vi "write_attributes.vi"(8 "error in (no error)":errorcluster, 10 "attributes":T1, 11 "GaussianNB in":refnum<class "GaussianNB.lvclass">) -> (0 "error out":errorcluster, 3 "GaussianNB out":refnum<class "GaussianNB.lvclass">)   [LabVIEW 2020, in "GaussianNB.lvclass"]
uses:
  GaussianNB.lvclass
  Controls/gaussian_nb_attributes.ctl
  GaussianNB.lvclass/GaussianNB.ctl
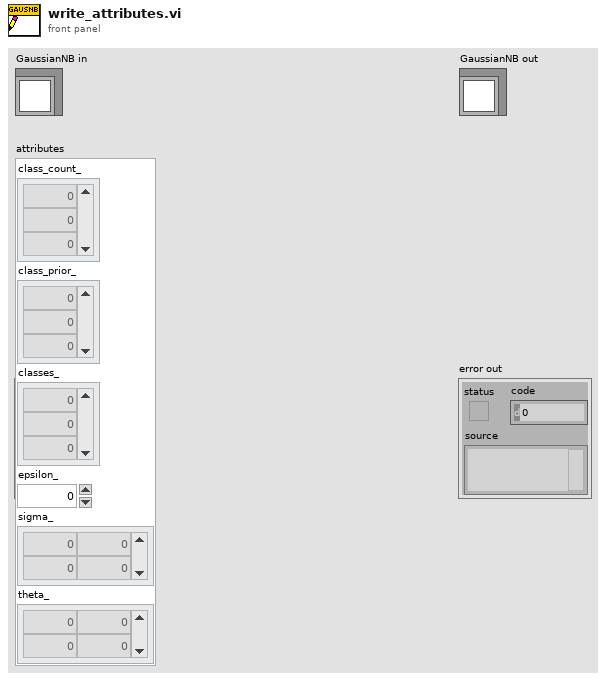
[diagram p1: front panel]
types:
  T1 = typedef "gaussian_nb_attributes.ctl" = cluster{"class_count_":dbl[], "class_prior_":dbl[], "classes_":dbl[], "epsilon_":dbl, "sigma_":dbl[][], "theta_":dbl[][]}
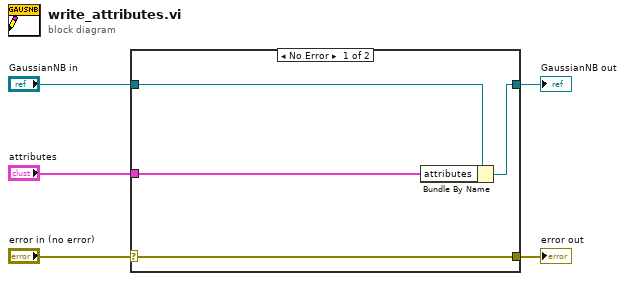
[diagram p0: block diagram]
diagram:
  n1 = case shown="No Error" "error in (no error)" {
    selector: "error in (no error)" -> [w9 w10]
    tunnel: [w9 w10] -> w4
    tunnel: [w7 w11] -> w2
    tunnel: "GaussianNB in" -> [w8 w11]
    tunnel: "attributes" -> [w6 _]
    frame No Error {
      n2 = Bundle By Name(cluster=w8, "attributes"=w6) -> (w7:refnum<class "GaussianNB.lvclass">)
    }
    frame Error {
    }
  }
  "error out" <- w4
  "GaussianNB out" <- w2
